vi "cm2nm_initialize_session_variables.vi"(2 "Session Name/ID_out":string, 3 "Notes_out":string, 4 "Instrument_out":u16, 5 "Session File_out":path) -> (0 "Fiducial Count":u32[](array[numeric]), 1 "Current Session Information":T1)   [LabVIEW 2011]
doc: "With information from the new session dialog, initialize the current session information."
uses:
  cm2nm_sample_set.ctl
  cm2nm_coordinate_information_v2.ctl
  Instrument_type_enum_v2.ctl
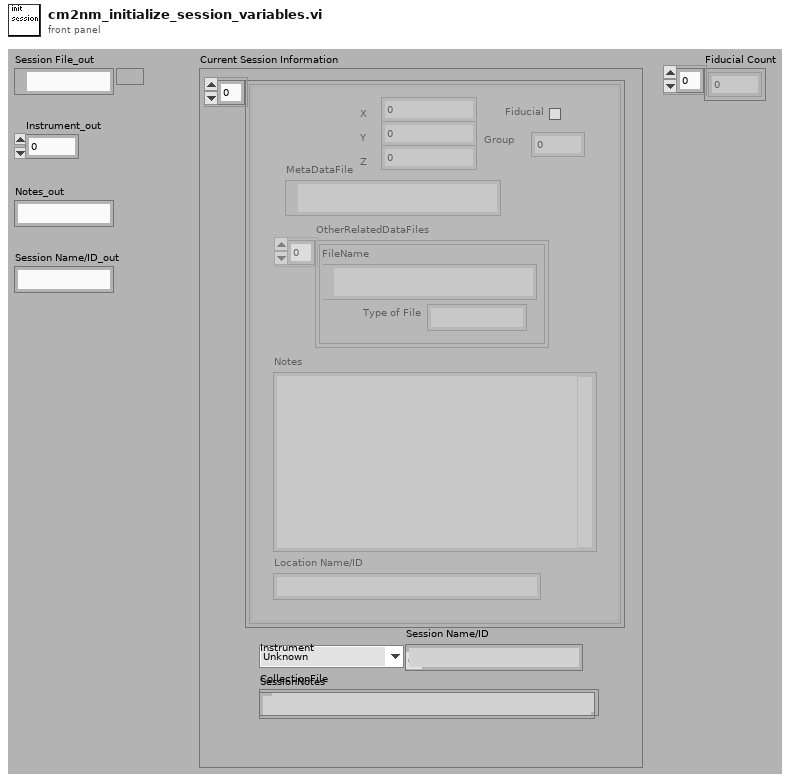
[diagram p1: front panel]
types:
  T1 = typedef "cm2nm_sample_set.ctl" = cluster{"CollectionOfPoints":T2[], "Instrument":T3, "CollectionFile":path, "Session Name/ID":string, "SessionNotes":string}
  T2 = typedef "cm2nm_coordinate_information_v2.ctl" = cluster{"MetaDataFile":path, "X":dbl, "Y":dbl, "Z":dbl, "Group":i32, "Rotation":dbl[unit], "Fiducial":bool, "Magnification":dbl, "Working_Distance":dbl, "Notes":string, "Location Name/ID":string, "OtherRelatedDataFiles":cluster{"Type of File":string, "FileName":path}[], "Available":bool}
  T3 = typedef "Instrument_type_enum_v2.ctl" = enum16{"Unknown", "Philips FEI SEM IRC", "JEOL 7000F EML_MFC", "MXRD MFC", "JEOL_EPMA"}
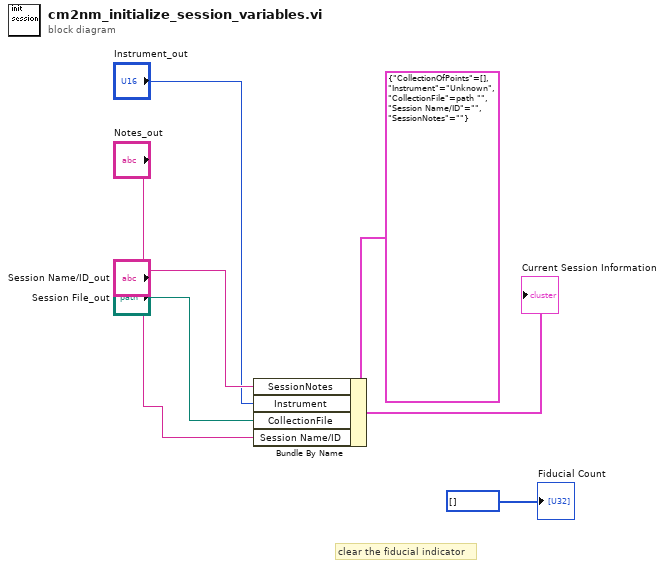
[diagram p0: block diagram]
diagram:
  # "clear the fiducial indicator"
  n1 = Bundle By Name(cluster=T1 {"CollectionOfPoints"=[], "Instrument"=enum."Unknown", "CollectionFile"=path "", "Session Name/ID"="", "SessionNotes"=""} ("Current Session Information"), "SessionNotes"="Notes_out", "Instrument"="Instrument_out", "CollectionFile"="Session File_out", "Session Name/ID"="Session Name/ID_out") -> (→"Current Session Information":T1)
  "Fiducial Count" <- u32[] [] ("Fiducial Count")
